vi "add.vi"() -> (3 "x+y":dbl)   [LabVIEW 2023]
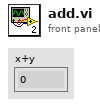
[diagram p1: front panel]
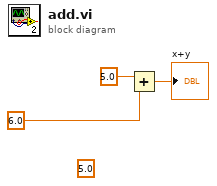
[diagram p0: block diagram]
diagram:
  (unwired) 5.0 ("y")
  n1 = Add(x=5.0, y=6.0) -> (x+y=→"x+y":dbl)
